vi "MT Detect CPM.vi"(5 "input complex waveform":T3={"t0"=0.0, "dt"=1.0, "Y"=[]} {"Y" format="%.3f"; "dt" format="%^.2e"; "t0" format="%.4f"}, 7 "CPM system parameters":T1={"samples per symbol (16)"=1, "symbol map"=[]}, 9 "synchronization parameters":T2 {"sync sequence" format="%.2f"}, 11 "error in (no error)":errorcluster, 12 "matched filter coefficients":dbl[](array[numeric]) format="%.2f", 13 "reset? (T)":bool=TRUE, 14 "flush buffers? (F)":bool) -> (6 "output bit stream":i8[](array[numeric]), 10 "sync found index (symbols)":dbl format="%.4f", 15 "error out":errorcluster)   [LabVIEW 2020, in "niDMT.lvlib"]
doc: "Demodulates a CPM-modulated complex baseband waveform and returns the demodulated information bit stream. This VI attempts to remove carrier and phase offset by locking to the carrier signal."
uses:
  <vilib>/addons/Modulation/niDMT.lvlib
  <vilib>/addons/Modulation/Analog/controls/Complex Data Waveform.ctl
  <vilib>/addons/Modulation/Digital/Support/Controls/CPM System Parameters.ctl
  <vilib>/Utility/error.llb/Error Cluster From Error Code.vi
  <vilib>/addons/Modulation/Digital/Support/Common/mod_Truncate FIR Filter (real).vi
  <vilib>/addons/Modulation/niAMT.lvlib
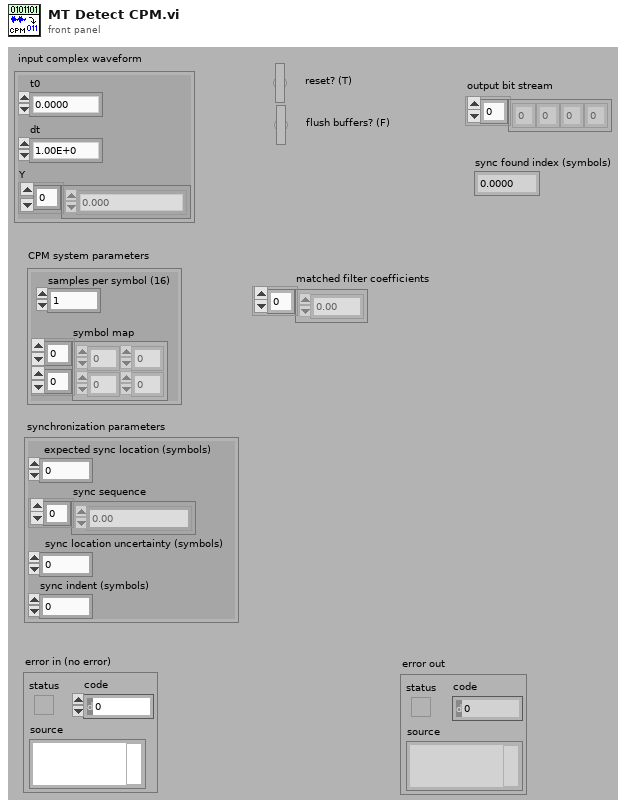
[diagram p1: front panel]
types:
  T1 = typedef "niDMT.lvlib/CPM System Parameters.ctl" = cluster{"samples per symbol (16)":i32, "symbol map":dbl[][]}
  T2 = cluster{"expected sync location (symbols)":i32, "sync sequence":cdb[], "sync location uncertainty (symbols)":i32, "sync indent (symbols)":i32}
  T3 = typedef "niAMT.lvlib/Complex Data Waveform.ctl" = cluster{"t0":dbl, "dt":dbl, "Y":cdb[]}
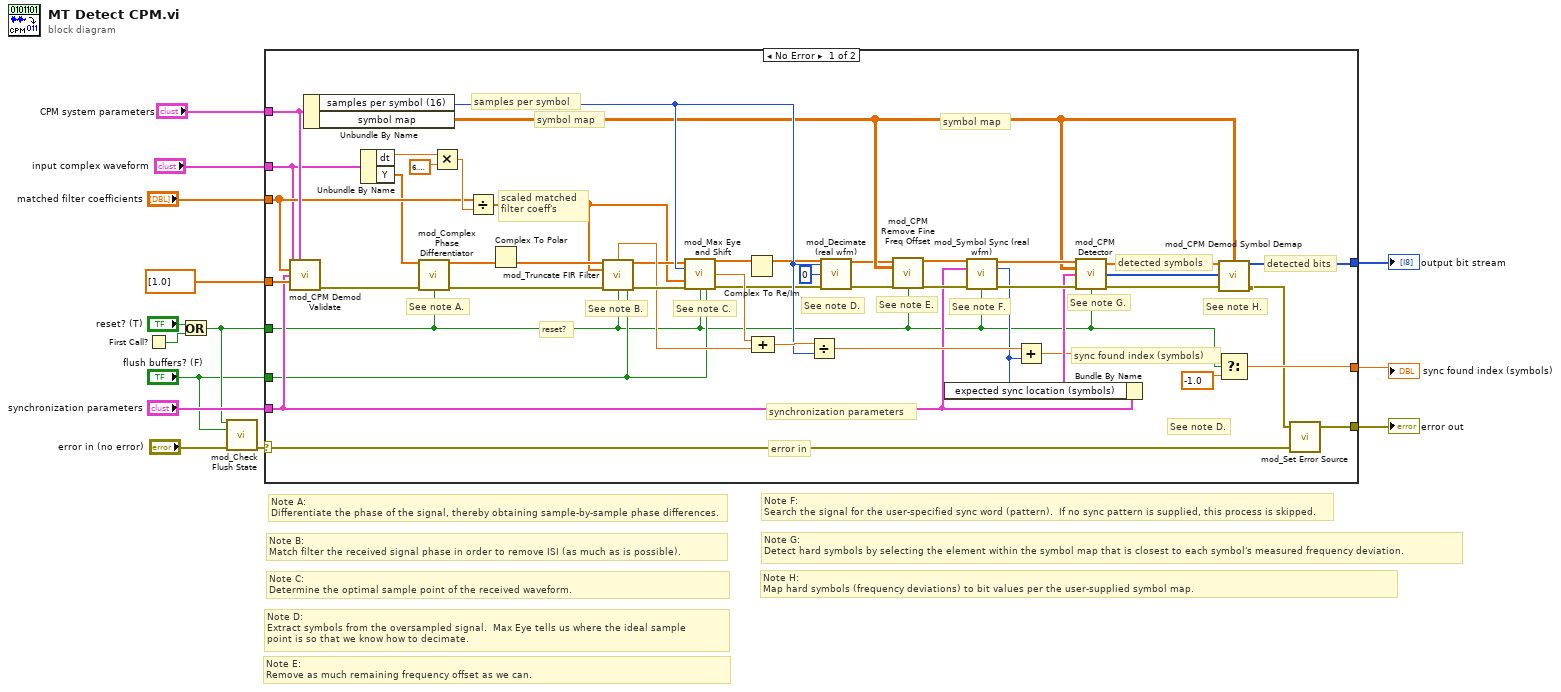
[diagram p0: block diagram]
diagram:
  # "Note H:\nMap hard symbols (frequency deviations) to bit values per the user-supplied symbol map."
  # "Note G:\nDetect hard symbols by selecting the element within the symbol map that is closest to each symbol's measured frequency deviation."
  # "Note F:\nSearch the signal for the user-specified sync word (pattern).  If no sync pattern is supplied, this process is skipped."
  # "Note E:\nRemove as much remaining frequency offset as we can."
  # "Note D:\nExtract symbols from the oversampled signal.  Max Eye tells us where the ideal sample \npoint is so that we know how to decimate."
  # "Note C:\nDetermine the optimal sample point of the received waveform."
  # "Note B:\nMatch filter the received signal phase in order to remove ISI (as much as is possible)."
  # "Note A:\nDifferentiate the phase of the signal, thereby obtaining sample-by-sample phase differences."
  n1 = First Call?() -> (First Call?: T/F=w6:bool)
  n2 = Or(x="reset? (T)", y=w6) -> (x .or. y?=w3:bool)
  n3 = call <vilib>:"mod_Check Flush State.vi"("reset?"=w3, "flush buffers? (F)"="flush buffers? (F)", "error in (no error)"="error in (no error)") -> ("error out"=w4:errorcluster)  [unwired: 12 out]
  n4 = case shown="No Error" w4 {
    selector: w4 -> [w57 w61]
    tunnel: [w58 w61] -> w9
    tunnel: "synchronization parameters" -> [w19 _]
    tunnel: "matched filter coefficients" -> [w42 _]
    tunnel: [w54 _] -> w10
    tunnel: "input complex waveform" -> [w41 _]
    tunnel: [w34 _] -> w11
    tunnel: w3 -> [w17 _]
    tunnel: "CPM system parameters" -> [w43 _]
    tunnel: dbl[] [1.0] ("Pulse Shaping Filter Coefficients") -> [w22 _]
    tunnel: "flush buffers? (F)" -> [w18 _]
    frame No Error {
      # "See note D."
      # "See note H."
      # "See note G."
      # "See note F."
      # "See note E."
      # "See note D."
      # "See note C."
      # "See note B."
      # "See note A."
      # "detected bits"
      # "error in"
      # "synchronization parameters"
      # "sync found index (symbols)"
      # "reset?"
      # "detected symbols"
      # "symbol map"
      # "scaled matched \nfilter coeff's"
      # "samples per symbol"
      # "symbol map"
      n5 = call <vilib>:"mod_CPM Demod Validate.vi"("Input Complex Waveform"=w41, "CPM system parameters"=w43, "Matched Filter Coefficients"=w42, "Synchronization Parameters"=w19, "Pulse Shaping Filter Coefficients"=w22) -> ("error out"=w40:errorcluster)  [unwired: 10 out]
      n6 = Unbundle By Name(w43) -> ("samples per symbol (16)"=w35:i32, "symbol map"=w27:dbl[][])
      n7 = Unbundle By Name(w41) -> ("dt"=w21:dbl, "Y"=w20:cdb[])
      n8 = call <vilib>:"mod_Complex Phase Differentiator.vi"("Signal In"=w20, "error in (no error)"=w40, "Reset? (T)"=w17) -> ("Signal Out"=w52:cdb[], "error out"=w46:errorcluster)  [unwired: 11 out]
      n9 = Multiply(x=w21, y=6.283185307179586) -> (x*y=w47:dbl)
      n10 = Divide(x=w42, y=w47) -> (x/y=w32:dbl[])
      n11 = Complex To Polar(r * e^(i*theta)=w52) -> (theta=w45:dbl[])  [unwired: 1 out]
      n12 = call-poly <vilib>:"mod_Truncate FIR Filter.vi"("Signal In"=w45, "Filter Coefficients"=w32, "error in (no error)"=w46, "Reset? (T)"=w17, "flush buffers? (F)"=w18) -> ("Fractional Delay (samples)"=w37:dbl, "Signal Out"=w33:dbl[], "error out"=w50:errorcluster)  [unwired: 8 out]
      n13 = call <vilib>:"mod_Max Eye and Shift.vi"("Signal In"=w33, "Samples Per Symbol (16)"=w35, "matched filter coefficients"=w32, "error in (no error)"=w50, "Reset? (T)"=w17, "flush buffers? (F)"=w18) -> ("Signal Out"=w16:cdb[], "Optimal Offset (in Samples)"=w31:dbl, "error out"=w30:errorcluster)  [unwired: 1 in, 6 out]
      n14 = Complex To Re/Im(x + iy=w16) -> (x=w15:dbl[])  [unwired: 1 out]
      n15 = Compound Arithmetic op=ADD(w31, w37) -> (w49:dbl)
      n16 = Divide(x=w49, y=w35) -> (x/y=w56:dbl)
      n17 = call <vilib>:"mod_Decimate (real wfm).vi"("Signal In"=w15, "Samples Per Symbol (16)"=w35, "Offset"=0, "error in (no error)"=w30) -> ("Signal Out"=w26:dbl[], "error out"=w25:errorcluster)  [unwired: 10 in]
      n18 = call <vilib>:"mod_CPM Remove Fine Freq Offset.vi"("Symbols"=w26, "Symbol Map"=w27, "error in (no error)"=w25, "Reset? (T)"=w17) -> ("Symbols"=w24:dbl[], "error out"=w23:errorcluster)  [unwired: 10 out]
      n19 = call <vilib>:"mod_Symbol Sync (real wfm).vi"("Signal In"=w24, "Synchronization Parameters"=w19, "error in (no error)"=w23, "Reset? (T)"=w17) -> ("Signal Out"=w51:dbl[], "Sync Location (symbols)"=w36:i32, "error out"=w60:errorcluster)  [unwired: 9 in]
      n20 = Bundle By Name(cluster=w19, "expected sync location (symbols)"=w36) -> (w59:T2)
      n21 = Add(x=w56, y=w36) -> (x+y=w53:dbl)
      n22 = call <vilib>:"mod_CPM Detector.vi"("Symbols"=w51, "Symbol Map"=w27, "Synchronization Parameters"=w59, "error in (no error)"=w60, "reset ? (T/F)"=w17) -> ("Detected Symbols"=w48:dbl[], "detected modulation indices"=w39:i32[], "error out"=w29:errorcluster)  [unwired: 8 out]
      n23 = call <vilib>:"mod_CPM Demod Symbol Demap.vi"("Symbols In"=w48, "Symbol Map"=w27, "input modulation indices"=w39, "error in (no error)"=w29) -> ("Bits Out"=w34:i8[], "error out"=w28:errorcluster)  [unwired: 1 in, 9 out]
      n24 = Select(t=w53, s=w17, f=-1.0) -> (s? t:f=w54:dbl)
      n25 = call <vilib>:"mod_Set Error Source.vi"("initial error in (no error)"=w57, "final error in (no error)"=w28) -> ("error out"=w58:errorcluster)  [unwired: 3 out]
    }
    frame Error {
    }
  }
  "error out" <- w9
  "sync found index (symbols)" <- w10
  "output bit stream" <- w11
